vi "ref_clock_out.vi"(6 "FPGA I/O":refnum<k21>="LED0", 11 "Half period":u16) -> (2 "Pos edge":bool)   [LabVIEW 2014]
uses:
  <vilib>/rvi/eio/common/nirviEmuTemplateMethod_errors.vi
  <vilib>/eio/EIONode/EIONode.xnode
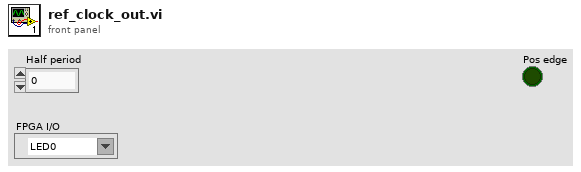
[diagram p1: front panel]
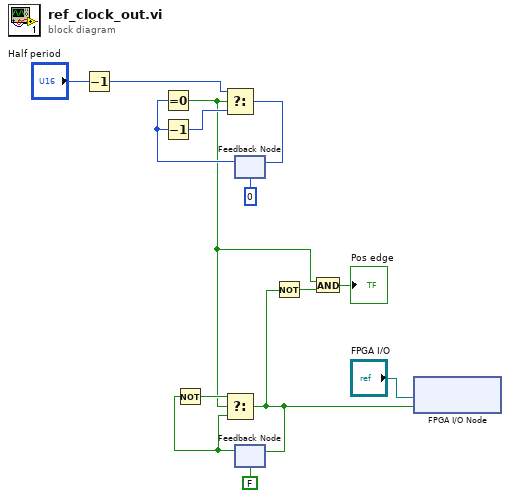
[diagram p0: block diagram]
diagram:
  n1 = Decrement(x="Half period") -> (x-1=w14:u16)
  n2 = feedback #1(u16 0 ("Numeric")) -> (w12:u16)
  n3 = Equal To 0?(x=w12) -> (x = 0?=w2:bool)
  n4 = Decrement(x=w12) -> (x-1=w10:u16)
  n5 = Select(t=w14, s=w2, f=w10) -> (s? t:f=w11:u16)
  n6 = feedback-in #1(w11) -> ()
  n7 = feedback #2(FALSE) -> (w8:bool)
  n8 = Not(x=w8) -> (.not. x?=w9:bool)
  n9 = Select(t=w9, s=w2, f=w8) -> (s? t:f=w1:bool)
  n10 = feedback-in #2(w1) -> ()
  n11 = Not(x=w1) -> (.not. x?=w4:bool)
  n12 = And(x=w2, y=w4) -> (x .and. y?=→"Pos edge":bool)
  n13 = xnode "FPGA I/O Node"("I/O Item"=w1, "FPGA I/O In"="FPGA I/O") -> ()  [unwired: 1 out]
